vi "Sinusoidal Move.vi"(6 "Cycle Count (0)":u32 max=4294967294, 7 "Period":dbl=0.2 min=0.2 max=429496729.5 step=0.1 format="%#.1f", 8 "error in (no error)":errorcluster, 9 "Device and Axis":string, 10 "Amplitude":i32, 11 "VISA resource name":refnum<visa-resource-name>) -> (0 "error out":errorcluster, 3 "VISA resource name out":refnum<visa-resource-name>)   [LabVIEW 2018, in "Zaber A Series.lvlib"]
doc: "Moves a device in a sinusoidal pattern. To define the sinusoidal motion parameters, specify the peak amplitude (half of the total amplitude) using device position units. You can optionally use the Convert Position Units to Device Units VI to convert from standard units of measure. Use a positive amplitude value to start at a negative peak and move forward, or a negative value to start at the positive peak and move backward. \n\nSpecify the period duration in milliseconds - period must be greater than zero. The period input has a resolution of 0.1ms.\n\nThe motion will end when a \"stop\" command or a \"move sin stop\" command is received, or when the optional cycle count has been reached.\n\nThis VI requires that the Initialize VI has been called with the same serial port. \n\nNote: See the Device Lookup control for the microstep size of your model, or check on the product specifications page for the product on www.zaber.com."
uses:
  Zaber A Series.lvlib
  Private/All Commands.ctl
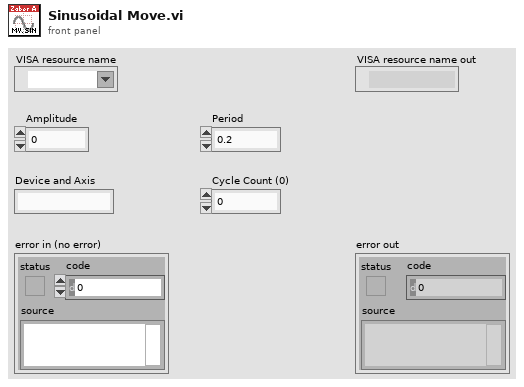
[diagram p1: front panel]
types:
  T1 = typedef "Zaber A Series.lvlib/All Commands.ctl" = string
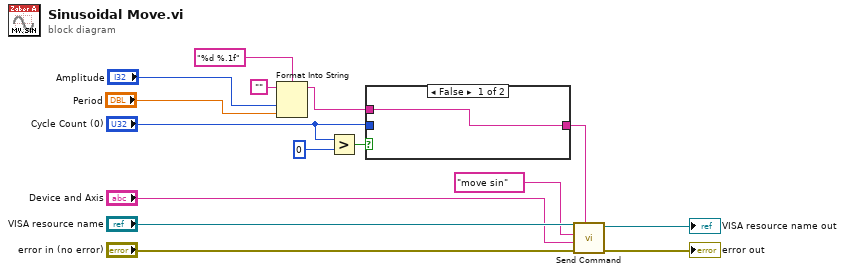
[diagram p0: block diagram]
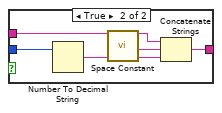
[diagram p2: hidden frame]
diagram:
  n1 = Format Into String(format string="%d %.1f", initial string="", "Amplitude", "Period") -> (resulting string=w6:string)  [unwired: 1 in, 1 out]
  n2 = Greater?(x="Cycle Count (0)", y=0) -> (0:w10:bool)
  n3 = case shown="False" w10 {
    tunnel: "Cycle Count (0)" -> [_ w21]
    tunnel: w6 -> [w16 w20]
    tunnel: [w16 w17] -> w8
    frame False {
    }
    frame True {
      n4 = Number To Decimal String(number=w21) -> (decimal integer string=w18:string)  [unwired: 1 in]
      n5 = call <vilib>:"Space Constant.vi"() -> ("String"=w19:string)
      n6 = Concatenate Strings(w20, w19, w18) -> (w17:string)
    }
  }
  n7 = call "Send Command.vi"("Data"=w8, "error in (no error)"="error in (no error)", "Device and Axis"="Device and Axis", "Command"=T1 "move sin" ("Complete Command List"), "VISA resource name"="VISA resource name") -> ("error out"=→"error out":errorcluster, "VISA resource name out"=→"VISA resource name out":refnum<visa-resource-name>)  [unwired: 1 in, 4 out]
